vi "DC Motor Control V2.vi"() -> ()   [LabVIEW 2013, in "LabVIEW Interface for Arduino.lvlib"]
doc: "An example that reads a user selectable analog input pin on the Arduino."
uses:
  <vilib>/LabVIEW Interface for Arduino/LabVIEW Interface for Arduino.lvlib
  <vilib>/LabVIEW Interface for Arduino/Type Defs/Pin Mode.ctl
panel:
  out "Actaul Speed":dbl
  in  "User Set Speed":u8
  in  "PWM1 Pin":u8
  in  "Stop":bool
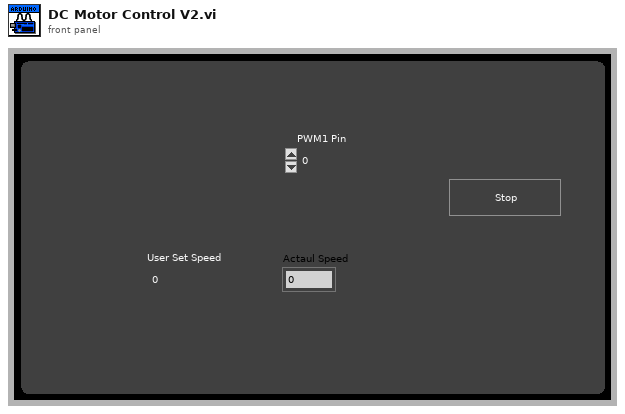
[diagram p1: front panel]
types:
  T1 = typedef "LabVIEW Interface for Arduino.lvlib/Pin Mode.ctl" = enum8{"Input", "Output"}
  T2 = typedef "LabVIEW Interface for Arduino.lvlib/Arduino Resource.ctl" = cluster{"VISA resource":refnum<visa-resource-name>, "Board Type":T3, "Connection Type":enum8{"USB / Serial"}, "Bytes Per Packet (15)":u8}
  T3 = typedef "LabVIEW Interface for Arduino.lvlib/Board Type.ctl" = enum16{"Uno", "Dimuelanove w/Atmega 328", "Mega 2560"}
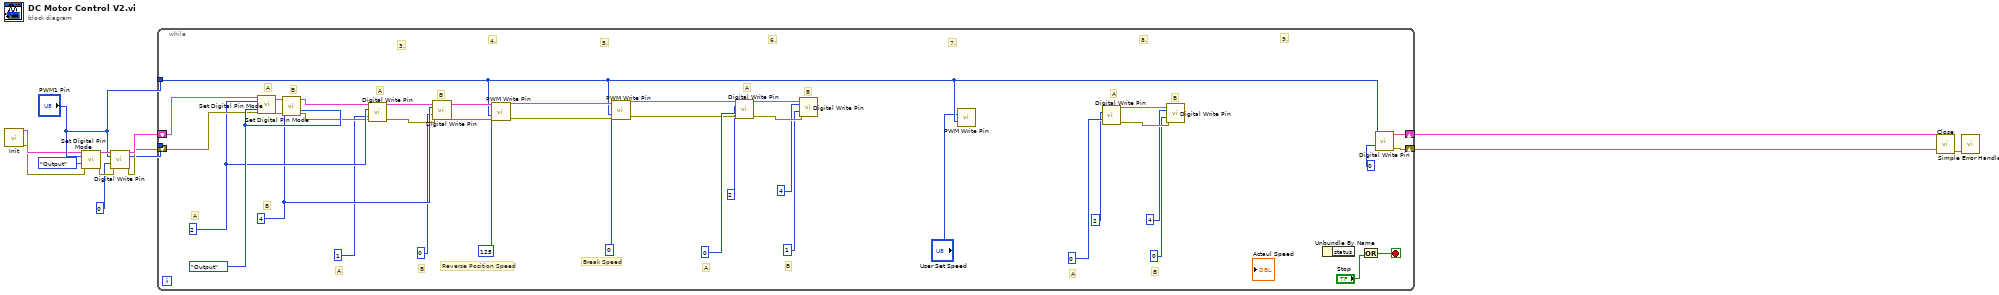
[diagram p0: block diagram]
diagram:
  n1 = call <vilib>:"Init.vi"() -> ("Arduino Resource"=w3:T2, "error out"=w2:errorcluster)  [unwired: 18 in]
  n2 = call <vilib>:"Set Digital Pin Mode.vi"("Arduino Resource"=w3, "Digital I/O Pin"="PWM1 Pin", "Pin Mode (Input)"=Pin_Mode."Output", "error in"=w2) -> ("Arduino Resource"=w9:T2, "error out"=w8:errorcluster)  [unwired: 10 in]
  n3 = call <vilib>:"Digital Write Pin.vi"("Arduino Resource"=w9, "Digital I/O Pin (0)"="PWM1 Pin", "Value (0)"=u8 0, "error in"=w8) -> ("Arduino Resource"=w6:T2, "error out"=w5:errorcluster)  [unwired: 10 in]
  n4 = while {
    shift-right: [w49] -> w11
    shift-left: w6 -> [w42]
    shift-right: [w48] -> w10
    shift-left: w5 -> [w41]
    tunnel: "PWM1 Pin" -> [_]
    tunnel: "PWM1 Pin" -> [w20]
    stop <- w52 stop-if-true
    w39 = u8 4 ("Digital I/O Pin")
    w40 = u8 2 ("Digital I/O Pin")
    w47 = Pin_Mode."Output" ("Pin Mode (Input)")
    # "9."
    # "8."
    # "B"
    # "A"
    # "B"
    # "A"
    # "7."
    # "6."
    # "B"
    # "A"
    # "B"
    # "A"
    # "Break Speed"
    # "5."
    # "4."
    # "Reverse Position Speed"
    # "3."
    # "B"
    # "A"
    # "B"
    # "A"
    # "B"
    # "A"
    # "B"
    # "A"
    n5 = call <vilib>:"Set Digital Pin Mode.vi"("Arduino Resource"=w42, "Digital I/O Pin"=w40, "Pin Mode (Input)"=w47, "error in"=w41) -> ("Arduino Resource"=w46:T2, "error out"=w45:errorcluster)  [unwired: 10 in]
    n6 = call <vilib>:"Set Digital Pin Mode.vi"("Arduino Resource"=w46, "Digital I/O Pin"=w39, "Pin Mode (Input)"=w47, "error in"=w45) -> ("Arduino Resource"=w38:T2, "error out"=w37:errorcluster)  [unwired: 10 in]
    n7 = call <vilib>:"Digital Write Pin.vi"("Arduino Resource"=w38, "Digital I/O Pin (0)"=w40, "Value (0)"=u8 1, "error in"=w37) -> ("Arduino Resource"=w44:T2, "error out"=w43:errorcluster)  [unwired: 10 in]
    n8 = call <vilib>:"Digital Write Pin.vi"("Arduino Resource"=w44, "Digital I/O Pin (0)"=w39, "Value (0)"=u8 0, "error in"=w43) -> ("Arduino Resource"=w34:T2, "error out"=w33:errorcluster)  [unwired: 10 in]
    n9 = call <vilib>:"PWM Write Pin.vi"("Arduino Resource"=w34, "Duty Cycle (0 - 255)"=u8 125, "PWM Pin (3)"=w20, "error in"=w33) -> ("Arduino Resource"=w30:T2, "error out"=w29:errorcluster)  [unwired: 10 in]
    n10 = call <vilib>:"PWM Write Pin.vi"("Arduino Resource"=w30, "Duty Cycle (0 - 255)"=u8 0, "PWM Pin (3)"=w20, "error in"=w29) -> ("Arduino Resource"=w24:T2, "error out"=w23:errorcluster)  [unwired: 10 in]
    n11 = call <vilib>:"Digital Write Pin.vi"("Arduino Resource"=w24, "Digital I/O Pin (0)"=u8 2, "Value (0)"=u8 0, "error in"=w23) -> ("Arduino Resource"=w28:T2, "error out"=w27:errorcluster)  [unwired: 10 in]
    n12 = call <vilib>:"Digital Write Pin.vi"("Arduino Resource"=w28, "Digital I/O Pin (0)"=u8 4, "Value (0)"=u8 1, "error in"=w27) -> ()  [unwired: 10 in, 2 out]
    n13 = call <vilib>:"PWM Write Pin.vi"("Duty Cycle (0 - 255)"="User Set Speed", "PWM Pin (3)"=w20) -> ()  [unwired: 12 in, 2 out]
    n14 = call <vilib>:"Digital Write Pin.vi"("Digital I/O Pin (0)"=u8 2, "Value (0)"=u8 0) -> ("Arduino Resource"=w18:T2, "error out"=w17:errorcluster)  [unwired: 12 in]
    n15 = call <vilib>:"Digital Write Pin.vi"("Arduino Resource"=w18, "Digital I/O Pin (0)"=u8 4, "Value (0)"=u8 0, "error in"=w17) -> ()  [unwired: 10 in, 2 out]
    n16 = Unbundle By Name() -> ()  [unwired: 1 in, 1 out]
    n17 = Or(y="Stop") -> (x .or. y?=w52:bool)  [unwired: 1 in]
    n18 = call <vilib>:"Digital Write Pin.vi"("Digital I/O Pin (0)"=w20, "Value (0)"=u8 0) -> ("Arduino Resource"=w49:T2, "error out"=w48:errorcluster)  [unwired: 12 in]
  }
  n19 = call <vilib>:"Close.vi"("Arduino Resource"=w11, "error in"=w10) -> ("error out"=w12:errorcluster)  [unwired: 13 in]
  n20 = call <vilib>:"Simple Error Handler.vi"("error in (no error)"=w12) -> ()  [unwired: 4 in, 5 out]
